vi "CH_LM Utility Probe Information.vi"(0 "Meter Index":i32, 2 "Read All Properties (T)":bool=TRUE, 5 "error in (no error)":errorcluster, 7 "Timeout / ms (3000)":i32=3000, 9 "Lock Timeout / ms (1000)":i32=1000) -> (8 "Probe Diameter":dbl[unit] format="%#.2g", 10 "Model":string, 11 "Lock timed out":bool, 12 "Probe Type":T2, 13 "Serial Number":string, 14 "Meter Index":i32, 15 "Probe Qualifier":T1, 16 "Calibration Date":timestamp format="%<%x>T", 17 "Head Temperature":dbl[unit]=273.15, 18 "Responsitivity":dbl format="%#.1g", 19 "error out":errorcluster)   [LabVIEW 2012, in "CH_LM.lvlib"]
doc: "This VI queries for probe information."
uses:
  CH_LM.lvlib
  CH_LM ProbeType.ctl
  CH_LM ProbeQualifier.ctl
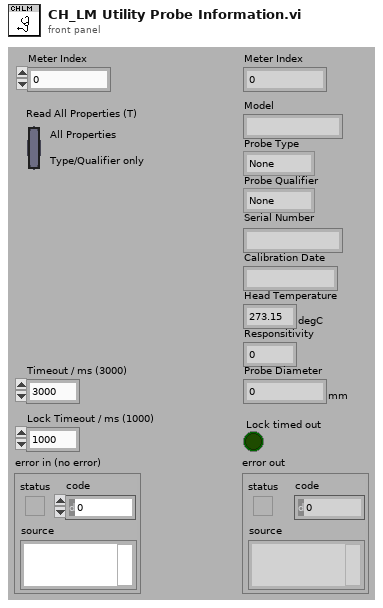
[diagram p1: front panel]
types:
  T1 = typedef "CH_LM.lvlib/CH_LM ProbeQualifier.ctl" = enum16{"None", "Single", "Quad", "No Spec"}
  T2 = typedef "CH_LM.lvlib/CH_LM ProbeType.ctl" = enum16{"None", "Thermopile", "Pyroelectric", "Optical"}
  T3 = cluster{"second":i32, "minute":i32, "hour":i32, "day of month":i32, "month":i32, "year":i32, "day of week":i32, "day of year":i32, "is DST":i32}
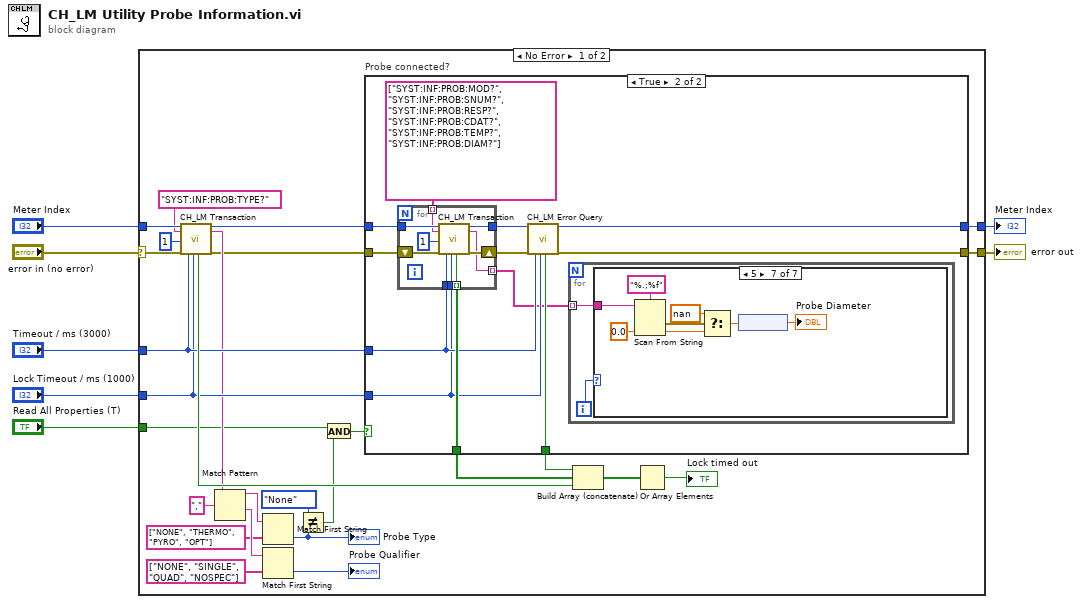
[diagram p0: block diagram]
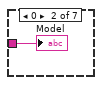
[diagram p4: hidden frame]
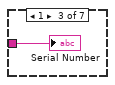
[diagram p5: hidden frame]
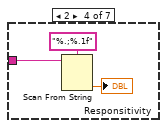
[diagram p6: hidden frame]
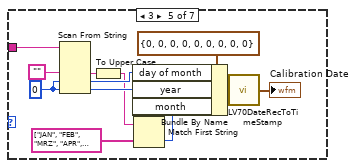
[diagram p7: hidden frame]
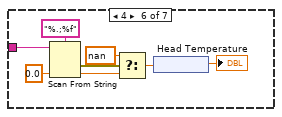
[diagram p8: hidden frame]
diagram:
  n1 = case shown="No Error" "error in (no error)" {
    selector: "error in (no error)" -> [w12 w95]
    tunnel: [w34 w95] -> w7
    tunnel: "Meter Index" -> [w26 w94]
    tunnel: [w33 w94] -> w4
    tunnel: "Timeout / ms (3000)" -> [w23 _]
    tunnel: "Lock Timeout / ms (1000)" -> [w22 _]
    tunnel: "Read All Properties (T)" -> [w10 _]
    frame No Error {
      n2 = call "CH_LM Transaction.vi"("Meter Index"=w26, "Command String"="SYST:INF:PROB:TYPE?", "NofStrings (-1:all)"=1, "error in (no error)"=w12, "Timeout / ms (3000)"=w23, "Lock Timeout / ms (1000)"=w22) -> ("Lock timed out"=w24:bool, "Meter Index"=w27:i32, "Response"=w15:string, "error out"=w11:errorcluster)  [unwired: 10 out]
      n3 = Match Pattern(string=w15, regular expression=",") -> (before substring=w17:string, after substring=w20:string)  [unwired: 3 out]
      n4 = Match First String(2:string[] ["NONE", "THERMO", "PYRO", "OPT"] ("string array"), 3:w17) -> (0:w13:i32)  [unwired: 1 out]
      "Probe Type" <- w13
      n5 = Match First String(2:string[] ["NONE", "SINGLE", "QUAD", "NOSPEC"] ("string array"), 3:w20) -> (0:→"Probe Qualifier":i32)  [unwired: 1 out]
      n6 = Not Equal?(x=CH_LM_ProbeType."None" ("Probe Type 2"), y=w13) -> (x != y?=w9:bool)
      n7 = And(x=w10, y=w9) -> (x .and. y?=w8:bool)
      n8 = case "Probe connected?" shown="True" w8 {
        tunnel: [w35 w48] -> w34
        tunnel: [w36 w47] -> w33
        tunnel: [_ w46] -> w32
        tunnel: [_ w42] -> w29
        tunnel: w11 -> [w35 w41]
        tunnel: w27 -> [w36 w40]
        tunnel: w23 -> [_ w39]
        tunnel: w22 -> [_ w38]
        frame False {
        }
        frame True {
          n9 = for {
            tunnel: [w91] -> w44
            tunnel: w40 -> [w90]
            tunnel: w39 -> [w89]
            tunnel: w38 -> [w88]
            tunnel: string[] ["SYST:INF:PROB:MOD?", "SYST:INF:PROB:SNUM?", "SYST:INF:PROB:RESP?", "SYST:INF:PROB:CDAT?", "SYST:INF:PROB:TEMP?", "SYST:INF:PROB:DIAM?"] -> [w87] mode=indexing
            tunnel: [w85] -> w42 mode=indexing
            shift-right: [w92] -> w45
            shift-left: w41 -> [w93]
            tunnel: [w84] -> w37 mode=indexing
            n10 = call "CH_LM Transaction.vi"("Meter Index"=w90, "Command String"=w87, "NofStrings (-1:all)"=1, "error in (no error)"=w93, "Timeout / ms (3000)"=w89, "Lock Timeout / ms (1000)"=w88) -> ("Lock timed out"=w85:bool, "Meter Index"=w91:i32, "Response"=w84:string, "error out"=w92:errorcluster)  [unwired: 10 out]
          }
          n11 = call "CH_LM Error Query.vi"("Meter Index"=w44, "error in (no error)"=w45, "Timeout / ms (3000)"=w39, "Lock Timeout / ms (1000)"=w38) -> ("Lock timed out"=w46:bool, "Meter Index"=w47:i32, "error out"=w48:errorcluster)  [unwired: 13 out]
          n12 = for {
            tunnel: w37 -> [w49] mode=indexing
            i -> [w50]
            n13 = case shown="5" w50 {
              tunnel: w49 -> [_ w51 w52 w55 w62 w75 w83]
              frame Default {
              }
              frame 0 {
                "Model" <- w51
              }
              frame 1 {
                "Serial Number" <- w52
              }
              frame 2 {
                n14 = Scan From String(format string="%.;%.1f", input string=w55) -> (output 1=→"Responsitivity":dbl)  [unwired: 2 in, 4 out]
              }
              frame 3 {
                w63 = 0
                n15 = Scan From String(input string=w62, default 1="", default 2=w63, default 3=w63) -> (output 1=w59:string, output 2=w61:i32, output 3=w60:i32)  [unwired: 3 in, 3 out]
                n16 = To Upper Case(1:w59) -> (0:w58:string)
                n17 = Match First String(2:string[] ["JAN", "FEB", "MRZ", "APR", "MAI", "JUN", "JUL", "AUG", "SEP", "OKT", "NOV", "DEZ"], 3:w58) -> (0:w57:i32)  [unwired: 1 out]
                n18 = Bundle By Name(cluster=T3 {"second"=0, "minute"=0, "hour"=0, "day of month"=0, "month"=0, "year"=0, "day of week"=0, "day of year"=0, "is DST"=0} ("date time rec"), "day of month"=w61, "year"=w60, "month"=w57) -> (w67:T3)
                n19 = call <vilib>:"LV70DateRecToTimeStamp.vi"("date time rec"=w67) -> ("Time Stamp"=→"Calibration Date":timestamp)
              }
              frame 4 {
                n20 = Scan From String(format string="%.;%f", input string=w75, default 1=0.0) -> (error out=w72:errorcluster, output 1=w71:dbl)  [unwired: 2 in, 2 out]
                n21 = Select(t=nan, s=w72, f=w71) -> (s? t:f=w70:dbl)
                n22 = node(w70) -> (→"Head Temperature":dbl[unit])
              }
              frame 5 {
                n23 = Scan From String(format string="%.;%f", input string=w83, default 1=0.0) -> (error out=w81:errorcluster, output 1=w80:dbl)  [unwired: 2 in, 2 out]
                n24 = Select(t=nan, s=w81, f=w80) -> (s? t:f=w79:dbl)
                n25 = node(w79) -> (→"Probe Diameter":dbl[unit])
              }
            }
          }
        }
      }
      n26 = Build Array (concatenate)(w32, w29, w24) -> (w31:bool[])
      n27 = Or Array Elements(Boolean array=w31) -> (logical OR=→"Lock timed out":bool)
    }
    frame Error {
    }
  }
  "error out" <- w7
  "Meter Index" <- w4
